vi "SubPanel_DataCollection_Rev11_v14.vi"(0 "DCPowerInformationClusterArray_Input":T6(array[cluster]), 1 "VISAPowerInfoInputArray":T5(array[cluster]), 2 "Run Data SubPanel Input":T4, 3 "RF Block Input Array":T1[](array[typedef]), 4 "Oscilloscope Info Array":T3(array[cluster]) {"vertical coupling" items=["AC", "DC", "Ground"]}, 5 "Plot Color Array":u32[](array[colorbox])=[16711686, 65351, 8978420, 14474240, 16139007, 16752640, 8958719, 16758973, 16777215, 46792, 11992992, 12961221, 16763690, 12600063, 16711835, 2953983, 40796, 13111296, 13352613, 9221011, 12964076, 12819897, 65442, 16776704, 14540253, 16740729, 10658047, 10813344, 16753521, 13413843, 8691115, 10339240, 14401205, 16746704, 7467519, 16775978, 13872558, 11387603, 13354405, 10420227, 13107364, 4060, 35208, 11817216, 7566080, 40796, 7539456, 2837073, 6372186, 7499083, 10648702, 16757152], 6 "New Run?":bool, 7 "error in":errorcluster) -> (20 "DCPowerInformationClusterArray_Output":T6(array[cluster]), 21 "VISAPowerInfoInputOutput":T5(array[cluster]), 22 "Run Data SubPanel Output":T4, 23 "RF Subpanel Output":T1[](array[typedef]), 24 "Oscilloscope Info Array Output":T3(array[cluster]) {"vertical coupling" items=["AC", "DC", "Ground"]}, 25 "Reinitialize?":bool, 26 "Data Was Collected?":bool, 27 "error out":errorcluster)   [LabVIEW 2019]
uses:
  Controls/DataBlockControl.ctl
  Controls/QueueDataControl_V3.ctl
  <vilib>/Utility/file.llb/Write Delimited Spreadsheet (string).vi
  Controls/RFBlockControl.ctl
  <instrlib>/niScope/Controls/niScope vertical coupling.ctl
panel:
  in  "Total Current Y Min":dbl
  in  "Total Current Y Max":dbl
  in  "Total Voltage Y Min":dbl
  in  "Total Voltage Y Max":dbl
  in  "Total Measurement Range Update":bool
  in  "Live Measurement Range Update":bool
  in  "Live Current Y Min":dbl
  in  "Live Current Y Max":dbl
  in  "Live Voltage Y Min":dbl
  in  "Live Voltage Y Max":dbl
  out "Current Measurements Live":cluster{dbl[], dbl[]}[](graph)
  out "Voltage Measurements Live":cluster{dbl[], dbl[]}[](graph)
  out "RFSourceInfoArray":string[][](array[string])
  out "OscilloscopeInfoArray":string[][](array[string])
  out "Voltage Waveform Array":waveform(dbl)[](graph)
  out "Current Waveform Array":waveform(dbl)[](graph)
  out "DCPowerInfoArray":string[][](array[string])
  out "Current Measurements Total":cluster{dbl[], dbl[]}[](graph)
  out "Voltage Measurements Total":cluster{dbl[], dbl[]}[](graph)
  out "Exiting":bool
  out "Full Run Information":string
  out "Ready For Next Run?":bool
  in  "Next Run":bool
  out "Recording Data":bool
  in  "Record Data Toggle":bool
  out "error of collection":errorcluster
  in  "force exit SubVI":bool
  out "RF Block Parameters Output":T1
  # "Background information (Important)\nThere are three sets of voltage/current graphs\n\nOne is live always and just shows what all the channels look like _______ Waveform Array\n\nOne is live when measuring and shows some duration of the recording _______ Measurements Live\n\nOne shows the entire duration of the run, but it will take a few seconds to compile, just be patient it will populate\n\n\nInstructions (More Important)"
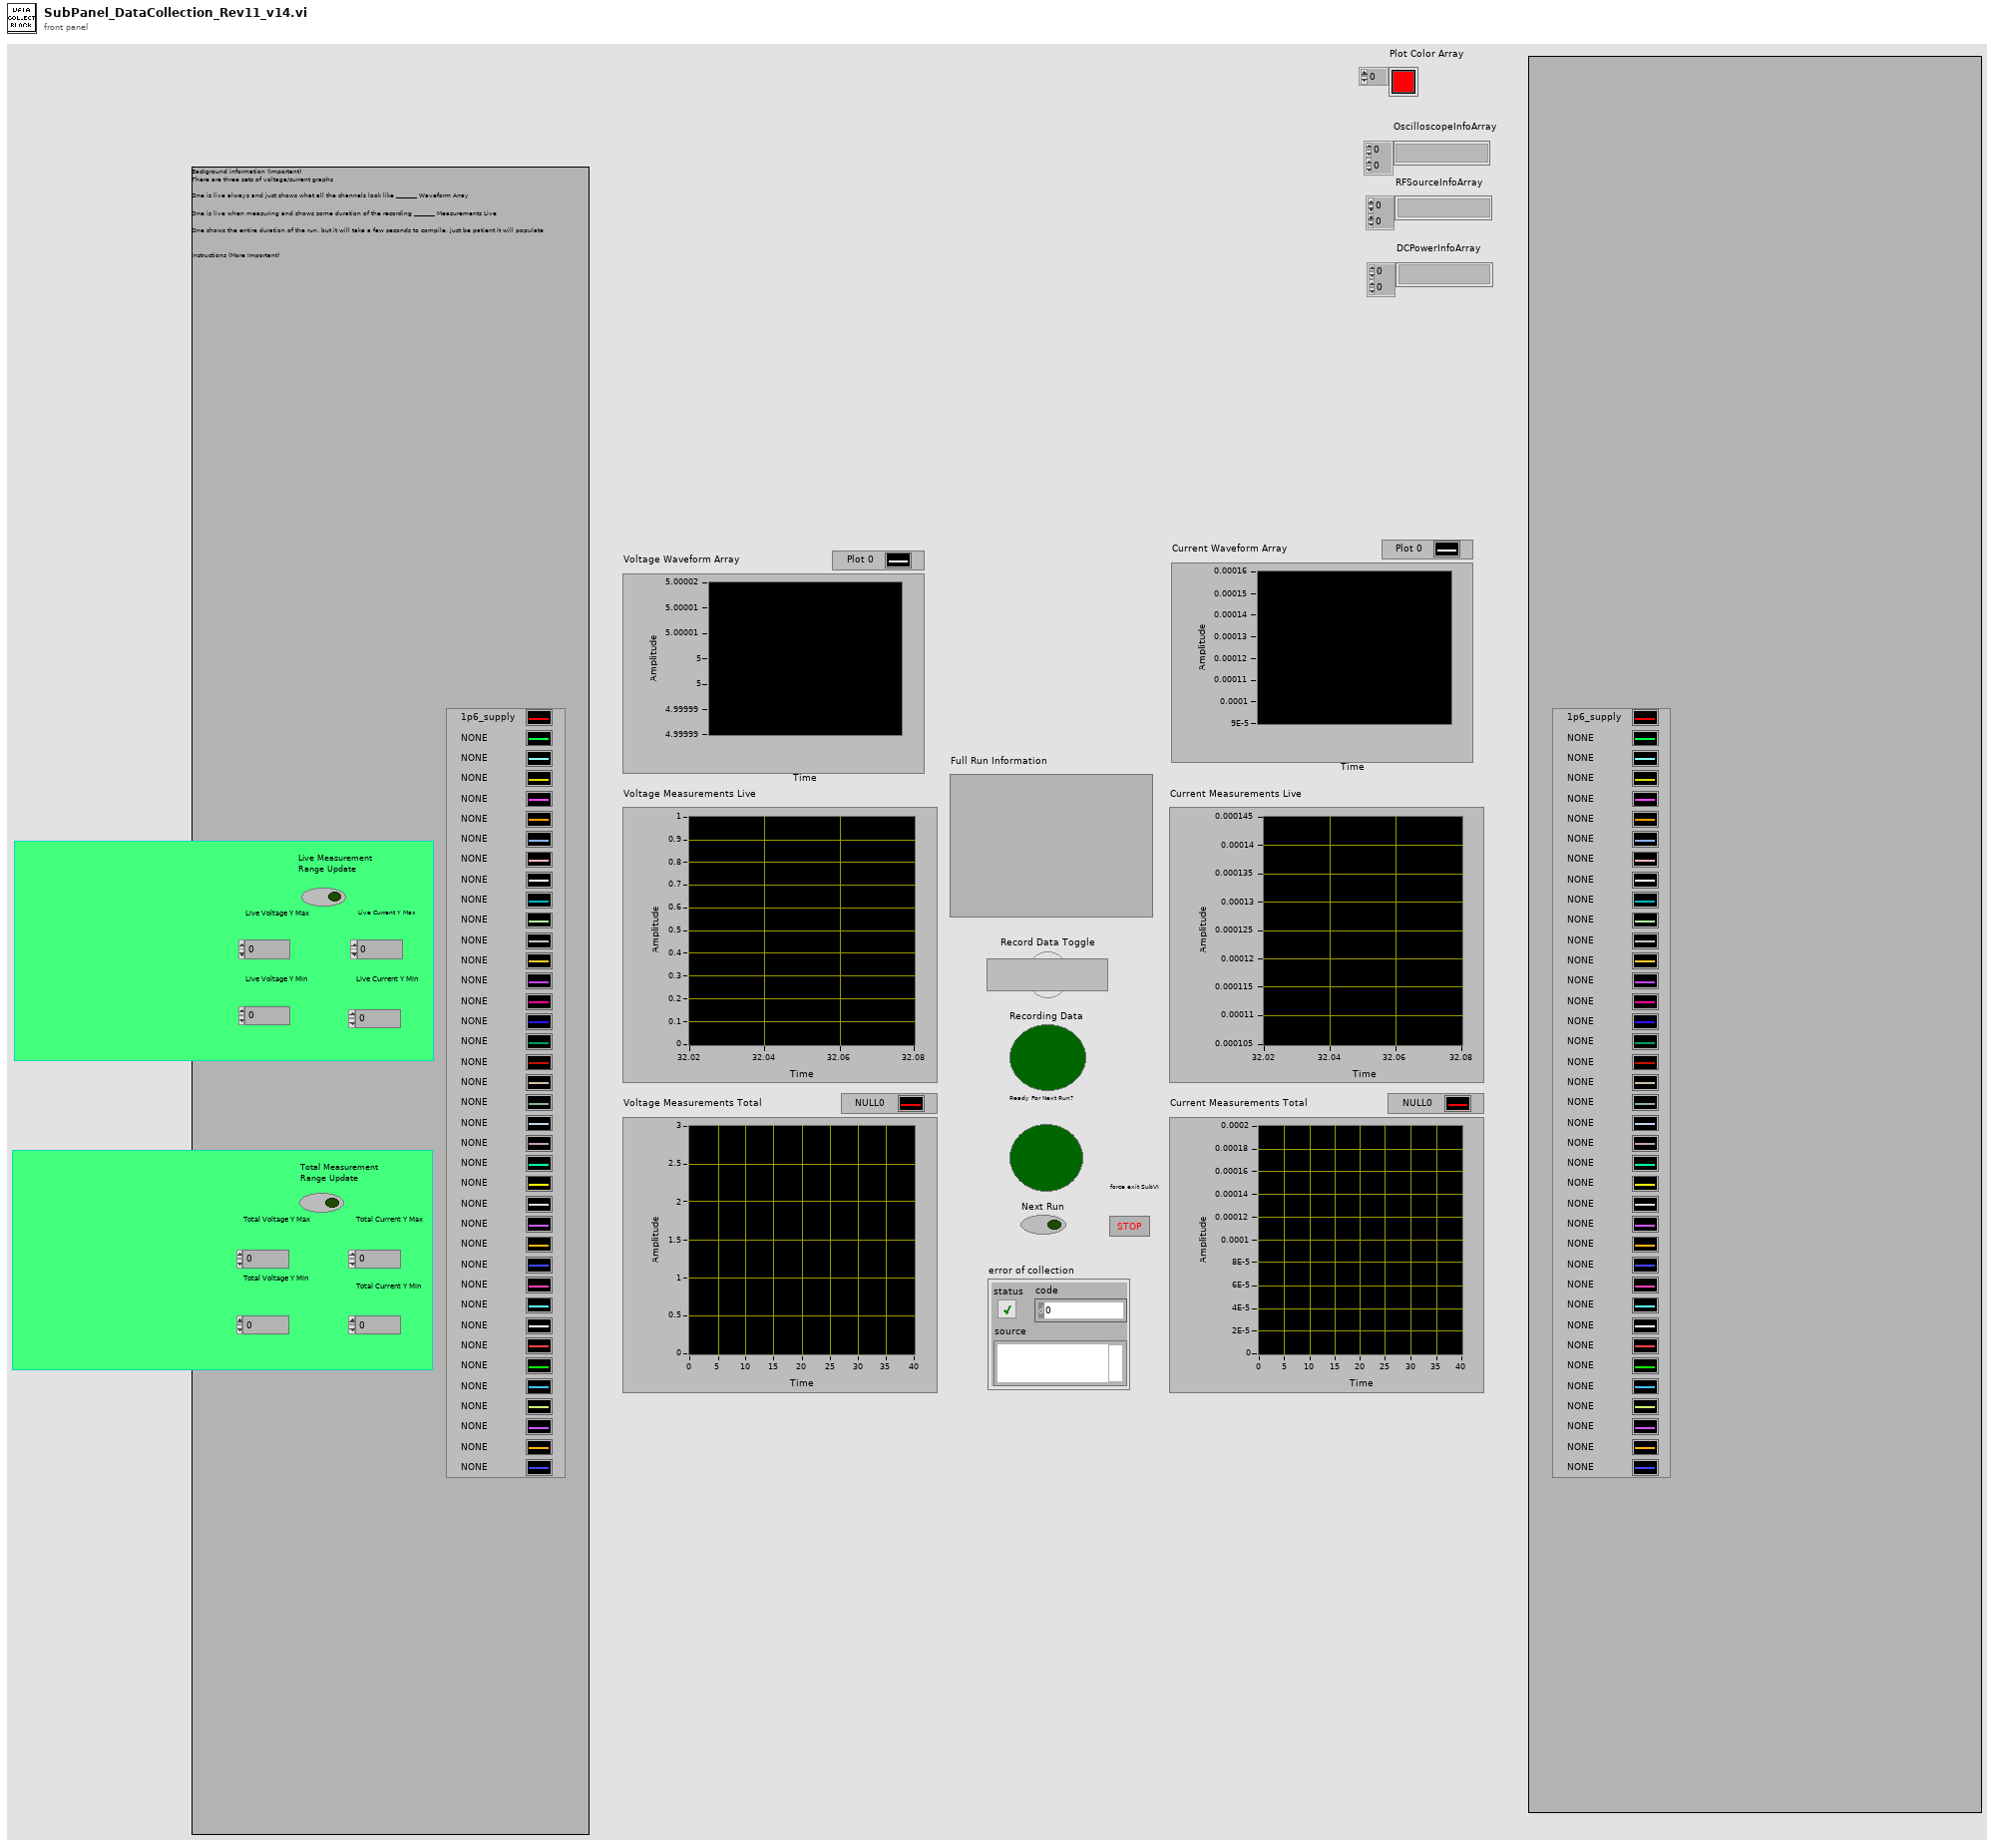
[diagram p1: front panel]
types:
  T1 = typedef "RFBlockControl.ctl" = cluster{"VISA resource name":refnum<visa-resource-name>, "RF Power State In":bool, "Frequency (GHz) Output":dbl, "Power (dBm) Output":dbl, "Instrument Name":string}
  T2 = typedef "niScope vertical coupling.ctl" = i32
  T3 = cluster{"instrument handle out":refnum<k15>, "channel numbers array":string[], "channel names array":string[], "vertical range":dbl, "vertical coupling":T2, "Channel 0 50 ohms?":bool, "50 ohm vertical range (V)":dbl, "min record length":i32, "Actual Sample Rate":dbl}[]
  T4 = typedef "DataBlockControl.ctl" = cluster{"Run Folder Parent Directory":path, "DUT":string, "Ion (ex Kr)":string, "Board Number":string, "Effective LET":string, "Test Type":enum16{"Single Event Latchup", "Single Event Transient", "Single Event Upset"}}
  T5 = cluster{"VISA resource name":refnum<visa-resource-name>, "String List":string, string[], "Input Array (Voltage,Current_Limit)":dbl[], "Input Array (Voltage,Current_Limit)":dbl[], "Channel Names":string[], "read buffer":string}[]
  T6 = cluster{"instrument handle out":refnum<k15>, string, string[], dbl[], string[], "Current Limit Output Array":dbl[], dbl[]}[]
  T7 = typedef "QueueDataControl_V3.ctl" = cluster{"Array of fetched data":dbl[][][], "Channel Names Array":string[], "Voltage Waveform Array":waveform(dbl)[], "Current Waveform Array":waveform(dbl)[], "Resetting Time":timestamp}
  T8 = cluster{"IVI Refnum out":refnum<k15>, string, "voltage level channel 23":dbl, "Channel Name 23":string, "Current Limit":dbl, "Measure Record dt":dbl, string}[]
  T9 = cluster{"created path":path, "DCPowerInformation_byChannel":cluster{"IVI Refnum out":refnum<k15>, string, "voltage level channel 23":dbl, "Channel Name 23":string, "Current Limit":dbl, "Measure Record dt":dbl, string}[], string[]}
  T10 = cluster{"Array of fetched data":dbl[][], string, i32[]}
  T11 = enum16{"open", "replace", "create", "open or create", "replace or create", "replace or create with confirmation"}
  T12 = enum16{"Single Event Latchup", "Single Event Transient", "Single Event Upset"}
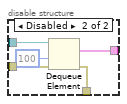
[diagram p5: hidden frame]
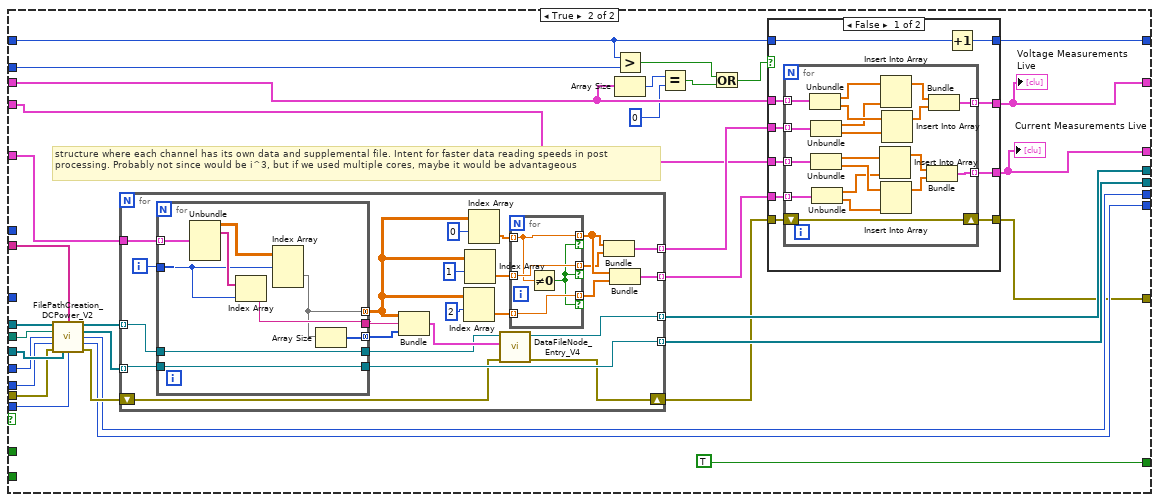
[diagram p7: hidden frame]
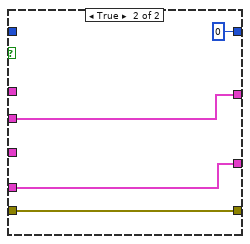
[diagram p8: hidden frame]
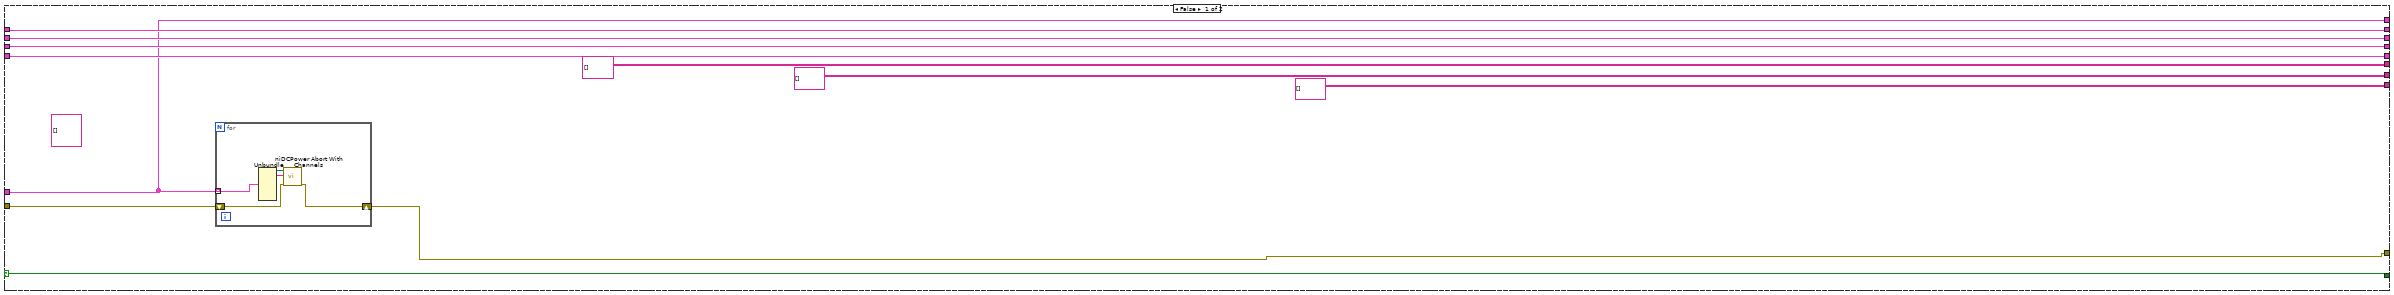
[diagram p9: hidden frame]
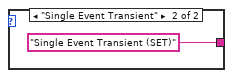
[diagram p10: hidden frame]
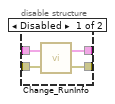
[diagram p14: hidden frame]
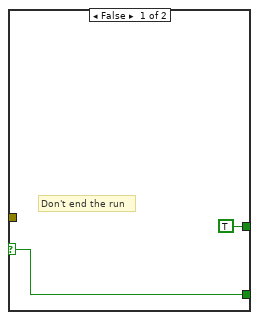
[diagram p17: hidden frame]
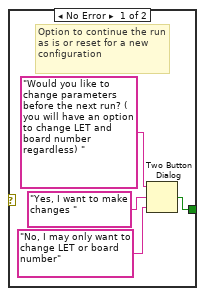
[diagram p18: hidden frame]
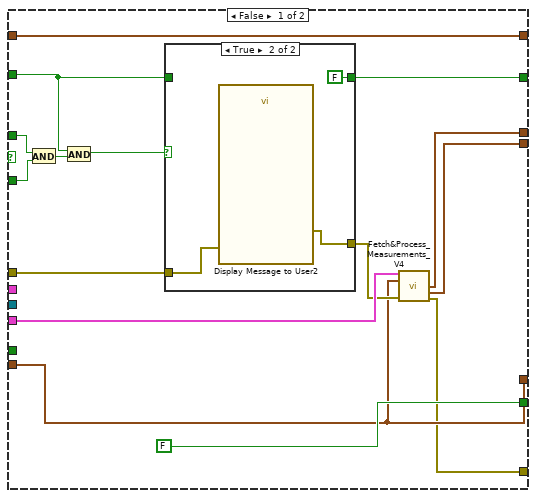
[diagram p20: hidden frame]
diagram:
  w15 = cluster{dbl[], dbl[]}[] [] ("array")
  (unwired) string[] ["Instrument Name", "Channel Name", "Instrument Channel Number", "Voltage (V)", "Current Limit (A)", "Measure Record delta Time (s)"] ("new element/subarray")
  w50 = T7 {"Array of fetched data"=[], "Channel Names Array"=[], "Voltage Waveform Array"=[], "Current Waveform Array"=[], "Resetting Time"=timestamp(0 s since 1904-01-01)} ("DCPower Queue Data Double Array Format")
  (unwired) T7 {"Array of fetched data"=[], "Channel Names Array"=[], "Voltage Waveform Array"=[], "Current Waveform Array"=[], "Resetting Time"=timestamp(0 s since 1904-01-01)} ("DCPower Double Array Queue")
  (unwired) 10000 ("binary file indexor in")
  (unwired) T4 {"Run Folder Parent Directory"=path "", "DUT"="", "Ion (ex Kr)"="", "Board Number"="", "Effective LET"="", "Test Type"=enum."Single Event Latchup"} ("Run Data Configuration")
  # "Need to make a function that will decrease the amount of loops if there are more channels active. Just exponential decay or a X/Y function but need some kind of offset which will probably be experimentally determined"
  # "Initiating the queue"
  # "echoing run information"
  # "Checking if this is a new run. If it is, a new folder is created along with references to a datafile node. If it is not new (i.e. you didn't start recording data because you needed to make a last minute change and pressed forced exit subvi), the previous folder that is theoretically empty (or just has the .txt files is used"
  # "If yes, you go into this subVI"
  # "This is the message at the beginning confirming if you want to make small changes to the program (i.e. LET)"
  # "Parameters from the configuration stage of this program"
  # "Reset the graph that is saving every 10 seconds of data. Every reset the low bound of the ten seconds is"
  # "Need to change to reflect number of channels that are being recorded. Collect this from a parameters file eventually that will be created"
  # "Indicator if the system is ready for another run. Also indicates if data was actually collected"
  # "Resets the system to start recording"
  # "A flag to ensure the warning message shows only once and doesn't lock the system"
  # "Initiating all of the DC Power instruments (doing this here so because we force abort channels in the DCPower setup because buffer overflow issues. Iterating over the instrument array and the active channel list"
  n1 = flat-sequence {
    tunnel: [w90] -> w66
    tunnel: "error in" -> [w80]
    tunnel: [w94] -> w71
    tunnel: "Run Data SubPanel Input" -> [w82]
    frame #0 {
      n2 = disable-structure shown="Enabled" {
        disable-tunnel: w80 -> [w97 w108]
        disable-tunnel: [w106 w108] -> w79
        frame Enabled {
          n3 = property on="Voltage Measurements Live" class="XYGraph (strict)"(error in=w97, "BG Color"=u32 0 ("Plot.Plot Color"), "Plot.Plot Interpolation"=u8 2) -> (error out=w96:errorcluster)  [unwired: 1 in, 1 out]
          n4 = property on="Current Measurements Live" class="XYGraph (strict)"(error in=w96, "BG Color"=u32 0 ("Plot.Plot Color"), "Plot.Plot Interpolation"=u8 2) -> (error out=w95:errorcluster)  [unwired: 1 in, 1 out]
          n5 = property on="Voltage Measurements Total" class="XYGraph (strict)"(error in=w95, "BG Color"=u32 0 ("Plot.Plot Color"), "Plot.Plot Interpolation"=u8 2) -> (error out=w107:errorcluster)  [unwired: 1 in, 1 out]
          n6 = property on="Current Measurements Total" class="XYGraph (strict)"(error in=w107, "BG Color"=u32 0 ("Plot.Plot Color"), "Plot.Plot Interpolation"=u8 2) -> (error out=w106:errorcluster)  [unwired: 1 in, 1 out]
        }
        frame Disabled {
        }
      }
      n7 = local write "Voltage Measurements Total"(cluster{dbl[], dbl[]}[] [] ("Voltage Measurements")) -> ()
      n8 = local write "Current Measurements Total"(cluster{dbl[], dbl[]}[] [] ("Current Measurements")) -> ()
      n9 = local write "Recording Data"(FALSE ("Recording Data")) -> ()
      n10 = local write "Exiting"(FALSE ("Forced Exit")) -> ()
      n11 = call "Convert_RunInfoCluster_2_RunInfoStringList.vi"("error in"=w79, "Run Number"="", "Run Data SubPanel Input"=w82) -> ("error output"=w83:errorcluster, "Run Data Output"=w84:string)
      n12 = call "Display Message to User"("error in (no error)"=w83, "Enable"=TRUE, "Message"=w84) -> ("error out"=w90:errorcluster)  [unwired: 7 in, 1 out]
      n13 = Two Button Dialog(message="Changing the LET?", 1:"No" ("F button name (\"Cancel\")"), 2:"Yes" ("T button name (\"OK\")")) -> (T button?=w94:bool)
    }
  }
  n14 = call "Convert_InstrumentReferenceArray_2_ChannelReferenceArray.vi"("error in (no error)"=w66, "DCPowerInformationClusterArray_Input"="DCPowerInformationClusterArray_Input") -> ("error out"=w65:errorcluster, "DCPowerInformation_byChannel"=w8:T8)
  n15 = case shown="True" w71 {
    tunnel: "Run Data SubPanel Input" -> [w110 w114]
    tunnel: [w110 w113] -> w24
    tunnel: [w109 w112] -> w67
    tunnel: w65 -> [w109 w111]
    frame False {
    }
    frame True {
      n16 = disable-structure shown="Enabled" {
        disable-tunnel: w114 -> [w118 w120]
        disable-tunnel: [w117 w119] -> w113
        disable-tunnel: [w116 w122] -> w112
        disable-tunnel: w111 -> [w115 w121]
        frame Disabled {
          n17 = call "Change_RunInfo.vi"("error in (no error)"=w115, "Run Data SubPanel in"=w118) -> ("error out"=w116:errorcluster, "Run Data SubPanel out"=w117:T4)
        }
        frame Enabled {
          n18 = call "Change_RunInfo_V2.vi"("error in (no error)"=w121, "Run Data SubPanel in"=w120) -> ("error out"=w122:errorcluster, "Run Data SubPanel out"=w119:T4)
        }
      }
    }
  }
  n19 = Unbundle(w24) -> ("Run Folder Parent Directory"=w68:path)  [unwired: 5 out]
  n20 = List Folder(path=w68, error in=w67) -> (folder names=w69:string[], error out=w53:errorcluster)  [unwired: 2 in, 2 out]
  n21 = Array Size(array=w69) -> (size(s)=w56:i32)
  n22 = case shown="True" "New Run?" {
    selector: "New Run?" -> [w124 w127]
    tunnel: [w125 w129] -> w57
    tunnel: w56 -> [w125 w128]
    tunnel: [w124 w127] -> w55
    tunnel: [w123 w126] -> w54
    tunnel: w53 -> [w123 w126]
    frame False {
    }
    frame True {
      n23 = Increment(x=w128) -> (x+1=w129:i32)
    }
  }
  n24 = Number To Decimal String(number=w57) -> (decimal integer string=w60:string)  [unwired: 1 in]
  n25 = Concatenate Strings("Run_", w60) -> (w23:string)
  n26 = Array Size(array=w8) -> (size(s)=w52:i32)
  n27 = call "InitialFileFolderCreation_V2.vi"("New Run?"=w55, "error in (no error)"=w54, "Run Number"=w23, "DCPowerArrayClusterSize"=w52, "base path"=w68) -> ("error out"=w22:errorcluster, "SupplementalDataFileReferenceObjectArray"=w63:refnum<file>[], "DataFileReferenceObjectArray"=w64:refnum<file>[], "created path"=w28:path)  [unwired: 3 in]
  n28 = call "Convert_RunInfoCluster_2_RunInfoStringList.vi"("error in"=w22, "Run Number"=w23, "Run Data SubPanel Input"=w24) -> ("error output"=w21:errorcluster, "Run Data Output"=→"Full Run Information":string)
  n29 = for {
    shift-right: [w130] -> w4
    shift-left: w21 -> [w132]
    tunnel: "DCPowerInformationClusterArray_Input" -> [w134] mode=indexing
    n30 = Unbundle(w134) -> ("instrument handle out"=w131:refnum<k15>, w133:string)  [unwired: 5 out]
    n31 = call <instrlib>:"niDCPower Initiate With Channels.vi"("error in (no error)"=w132, "channel name"=w133, "instrument handle"=w131) -> ("error out"=w130:errorcluster)  [unwired: 7 in, 1 out]
  }
  n32 = for {
    shift-right: [w137] -> w6
    shift-left: w4 -> [w139]
    tunnel: "Plot Color Array" -> [_] mode=indexing
    i -> [w135]
    w136 = "NONE" ("Plot.Plot Name")
    n33 = property on="Current Measurements Live" class="XYGraph (strict)"(error in=w139, "Active Plot"=w135, "Plot.Plot Name"=w136) -> (error out=w138:errorcluster)  [unwired: 1 in, 1 out]
    n34 = property on="Voltage Measurements Live" class="XYGraph (strict)"(error in=w138, "Active Plot"=w135, "Plot.Plot Name"=w136) -> (error out=w137:errorcluster)  [unwired: 1 in, 1 out]
  }
  n35 = case shown="Error .." w6 {
    selector: w6 -> [w140 _]
    tunnel: [w140 w141] -> w5
    tunnel: w4 -> [_ w141]
    frame No Error {
    }
    frame Error {
    }
  }
  n36 = for {
    tunnel: w8 -> [w144] mode=indexing
    tunnel: [w147] -> w9 mode=indexing
    shift-right: [w143] -> w11
    shift-left: w5 -> [w146]
    tunnel: "Plot Color Array" -> [w142] mode=indexing
    i -> [w148]
    # "Creating Array of Channel Names"
    n37 = Unbundle(w144) -> ("Channel Name 23"=w147:string)  [unwired: 6 out]
    n38 = property on="Current Measurements Live" class="XYGraph (strict)"(error in=w146, "Active Plot"=w148, "Plot.Plot Name"=w147, "Plot.Plot Color"=w142) -> (error out=w145:errorcluster)  [unwired: 1 in, 1 out]
    n39 = property on="Voltage Measurements Live" class="XYGraph (strict)"(error in=w145, "Active Plot"=w148, "Plot.Plot Name"=w147, "Plot.Plot Color"=w142) -> (error out=w143:errorcluster)  [unwired: 1 in, 1 out]
  }
  n40 = disable-structure shown="Enabled" {
    disable-tunnel: w11 -> [w152 w154]
    disable-tunnel: [w151 w154] -> w10
    disable-tunnel: [w150 _] -> w12
    disable-tunnel: w50 -> [w149 _]
    frame Enabled {
      n41 = Obtain Queue(name (unnamed)="DCPowerQueue", element data type=w149, error in (no error)=w152) -> (queue out=w150:refnum<queue>, error out=w151:errorcluster)  [unwired: 2 in, 1 out]
    }
    frame Disabled {
    }
  }
  n42 = Bundle("created path"=w28, "DCPowerInformation_byChannel"=w8, w9) -> (w42:T9)  [unwired: 1 in]
  n43 = Array Size(array=w9) -> (size(s)=w14:i32)
  n44 = Get Date/Time In Seconds() -> (seconds since 1Jan1904=w26:timestamp)
  n45 = while {
    tunnel: w12 -> [w194]
    shift-right: [w155] -> w47
    shift-left: w10 -> [w193]
    tunnel: w28 -> [w190]
    shift-right: [w183] -> w49
    shift-left: w64 -> [w191]
    shift-right: [w182] -> w48
    shift-left: w63 -> [w189]
    shift-right: [w185] -> _
    shift-left: 0 ("binary file indexor in") -> [w188]
    shift-right: [w184] -> _
    shift-left: 0 ("binary file indexor in") -> [w187]
    tunnel: 1000 ("binary file indexor in") -> [w186]
    tunnel: w9 -> [w192]
    tunnel: w14 -> [w161]
    shift-right: [w171] -> _
    shift-left: FALSE -> [w170]
    shift-right: [w167] -> _
    shift-left: 0 -> [w168]
    shift-right: [w166] -> _
    shift-left: w15 -> [w163]
    shift-right: [w165] -> _
    shift-left: w15 -> [w164]
    tunnel: 251 ("y") -> [w162]
    tunnel: "Plot Color Array" -> [w160]
    stop <- w179 stop-if-true
    # "If recording data is on, there should always be elements in the queue, so I shouldn't have to worry about a state where the \"recording data\" is active but there is no data in the queue, if so, then I'll just have to find an alternative to the OR statement"
    n46 = Get Queue Status(queue=w194, error in (no error)=w193) -> (queue out=w176:refnum<queue>, error out=w177:errorcluster, # elements in queue=w172:i32)  [unwired: 1 in, 5 out]
    n47 = local read "Recording Data"() -> (w169:bool)
    n48 = disable-structure shown="Enabled" {
      disable-tunnel: [w214 w216] -> w178
      disable-tunnel: w177 -> [w213 w218]
      disable-tunnel: w176 -> [w212 w219]
      disable-tunnel: [w211 w215] -> w175
      frame Enabled {
        n49 = Flush Queue(queue=w212, error in (no error)=w213) -> (remaining elements=w211:T7[], error out=w214:errorcluster)  [unwired: 1 out]
      }
      frame Disabled {
        n50 = Dequeue Element(queue=w219, timeout in ms (-1)=100, error in (no error)=w218) -> (element=w215:T7, error out=w216:errorcluster)  [unwired: 2 out]
      }
    }
    n51 = Not Equal To 0?(x=w172) -> (x != 0?=w174:bool)
    n52 = And(x=w174, y=w169) -> (x .and. y?=w173:bool)
    n53 = case shown="False" w173 {
      tunnel: w175 -> [_ w291]
      tunnel: w178 -> [w229 w285]
      tunnel: w192 -> [w230 w278]
      tunnel: w191 -> [w237 w290]
      tunnel: w190 -> [w231 w289]
      tunnel: w189 -> [w238 w288]
      tunnel: w188 -> [w236 w287]
      tunnel: w187 -> [w235 w277]
      tunnel: w186 -> [_ w276]
      tunnel: [w236 w284] -> w185
      tunnel: [w235 w283] -> w184
      tunnel: [w237 w280] -> w183
      tunnel: [w238 w279] -> w182
      tunnel: [w228 w270] -> w159
      tunnel: [w227 TRUE] -> w171
      tunnel: w170 -> [w226 _]
      tunnel: w169 -> [w234 _]
      tunnel: w168 -> [w225 w268]
      tunnel: [w224 w267] -> w167
      tunnel: [w223 w274] -> w166
      tunnel: [w222 w271] -> w165
      tunnel: w164 -> [w222 w266]
      tunnel: w163 -> [w223 w265]
      tunnel: w162 -> [_ w259]
      tunnel: w161 -> [w221 _]
      tunnel: w160 -> [w220 _]
      frame False {
        n54 = Not(x=w234) -> (.not. x?=w233:bool)
        n55 = And(x=w233, y=w226) -> (x .and. y?=w232:bool)
        n56 = case shown="True" w232 {
          tunnel: w231 -> [_ w253]
          tunnel: w230 -> [_ w252]
          tunnel: w229 -> [w241 w245]
          tunnel: [w241 w250] -> w228
          tunnel: [w240 FALSE] -> w227
          tunnel: w226 -> [w240 _]
          tunnel: w225 -> [w239 _]
          tunnel: [w239 0] -> w224
          tunnel: w221 -> [_ w243]
          tunnel: w220 -> [_ w242]
          frame False {
          }
          frame True {
            n57 = for {
              N: w243 -> [_]
              shift-right: [w256] -> w244
              shift-left: w245 -> [w257]
              tunnel: w242 -> [w254] mode=indexing
              i -> [w255]
              n58 = property on="Current Measurements Total" class="XYGraph (strict)"(error in=w257, "Active Plot"=w255, "Plot.Plot Color"=w254) -> (error out=w258:errorcluster)  [unwired: 1 in, 1 out]
              n59 = property on="Voltage Measurements Total" class="XYGraph (strict)"(error in=w258, "Active Plot"=w255, "Plot.Plot Color"=w254) -> (error out=w256:errorcluster)  [unwired: 1 in, 1 out]
            }
            n60 = call "ReadDataFile_V1.vi"("error in (no error)"=w244, "Create CSV files?"=FALSE, "Channel Names Array"=w252, "DataFolder Path"=w253) -> ("error out"=w250:errorcluster, "Current Measurements"=→"Current Measurements Total":cluster{dbl[], dbl[]}[], "Voltage Measurements"=→"Voltage Measurements Total":cluster{dbl[], dbl[]}[])  [unwired: 5 in]
          }
        }
      }
      frame True {
        # "structure where each channel has its own data and supplemental file. Intent for faster data reading speeds in post processing. Probably not since would be i^3, but if we used multiple cores, maybe it would be advantageous"
        n61 = call "FilePathCreation_DCPower_V2.vi"("binary file input reference array 1"=w290, "Channel Name Input array"=w278, "data output directory folder"=w289, "binary file indexor in"=w287, "Reset counter in"=w277, "error in (no error)"=w285, "binary file input reference array 2"=w288, "reset threshold"=w276) -> ("binary file output reference array"=w282:refnum<file>[], "binary file output reference array 2"=w281:refnum<file>[], "binary file indexor out"=w284:i32, "reset counter out"=w283:i32, "error out"=w286:errorcluster)  [unwired: 3 in]
        n62 = for {
          shift-right: [w338] -> w269
          shift-left: w286 -> [w339]
          tunnel: w291 -> [w348]
          tunnel: w281 -> [w345] mode=indexing
          tunnel: w282 -> [w344] mode=indexing
          tunnel: [w343] -> w279 mode=indexing
          tunnel: [w337] -> w280 mode=indexing
          tunnel: [w326] -> w273 mode=indexing
          tunnel: [w325] -> w272 mode=indexing
          i -> [w342]
          n63 = for {
            tunnel: w348 -> [w361] mode=indexing
            tunnel: w342 -> [w358]
            tunnel: [w353] -> w333 mode=concatenating
            tunnel: [w357] -> w347
            tunnel: w345 -> [w356]
            tunnel: w344 -> [w354]
            tunnel: [w354] -> w340
            tunnel: [w356] -> w343
            tunnel: [w355] -> w346 mode=concatenating
            n64 = Unbundle(w361) -> ("Array of fetched data"=w360:dbl[][][], "Channel Names Array"=w359:string[])  [unwired: 3 out]
            n65 = Index Array(array=w359, index=w358) -> (element=w357:string)
            n66 = Index Array(array=w360, index (dim 0)=w358) -> (element=w353:dbl[][])  [unwired: 2 in]
            n67 = Array Size(array=w353) -> (size(s)=w355:i32[])
          }
          n68 = Bundle("Array of fetched data"=w333, w347, w346) -> (w341:T10)  [unwired: 1 in]
          n69 = Index Array(array=w333, index (row)=2) -> (element=w330:dbl[])  [unwired: 1 in]
          n70 = Index Array(array=w333, index (row)=1) -> (element=w331:dbl[])  [unwired: 1 in]
          n71 = Index Array(array=w333, index (row)=0) -> (element=w332:dbl[])  [unwired: 1 in]
          n72 = call "DataFileNode_Entry_V4.vi"("error in (no error)"=w339, "Queued Elements"=w341, "Byte Stream File in"=w340) -> ("error out"=w338:errorcluster, "Byte Stream File out"=w337:refnum<file>)  [unwired: 7 in]
          n73 = for {
            tunnel: [w350] -> w329 mode=indexing if=w349
            tunnel: w332 -> [w350] mode=indexing
            tunnel: [w352] -> w327 mode=indexing if=w349
            tunnel: w331 -> [w352] mode=indexing
            tunnel: [w351] -> w328 mode=indexing if=w349
            tunnel: w330 -> [w351] mode=indexing
            n74 = Not Equal To 0?(x=w350) -> (x != 0?=w349:bool)
          }
          n75 = Bundle(w329, w327) -> (w326:cluster{dbl[], dbl[]})  [unwired: 1 in]
          n76 = Bundle(w329, w328) -> (w325:cluster{dbl[], dbl[]})  [unwired: 1 in]
        }
        n77 = Greater?(x=w268, y=w259) -> (0:w261:bool)
        n78 = Array Size(array=w265) -> (size(s)=w264:i32)
        n79 = Equal?(x=w264, y=0) -> (x = y?=w262:bool)
        n80 = Or(x=w261, y=w262) -> (x .or. y?=w260:bool)
        n81 = case shown="False" w260 {
          tunnel: [w297 w321] -> w274
          tunnel: w265 -> [w301 _]
          tunnel: w273 -> [w300 w321]
          tunnel: w266 -> [w299 _]
          tunnel: w272 -> [w298 w322]
          tunnel: [w296 w322] -> w271
          tunnel: [w295 w324] -> w270
          tunnel: w269 -> [w294 w324]
          tunnel: w268 -> [w293 _]
          tunnel: [w292 0] -> w267
          frame False {
            n82 = for {
              tunnel: w301 -> [w320] mode=indexing
              tunnel: w300 -> [w317] mode=indexing
              tunnel: w299 -> [w314] mode=indexing
              tunnel: w298 -> [w313] mode=indexing
              tunnel: [w304] -> w297 mode=indexing
              tunnel: [w303] -> w296 mode=indexing
              shift-right: [w302] -> w295
              shift-left: w294 -> [w302]
              n83 = Unbundle(w320) -> (w319:dbl[], w318:dbl[])
              n84 = Unbundle(w317) -> (w316:dbl[], w315:dbl[])
              n85 = Unbundle(w314) -> (w312:dbl[], w311:dbl[])
              n86 = Unbundle(w313) -> (w310:dbl[], w309:dbl[])
              n87 = Insert Into Array(array=w312, new element=w310) -> (w307:dbl[])  [unwired: 1 in]
              n88 = Insert Into Array(array=w319, new element=w316) -> (w305:dbl[])  [unwired: 1 in]
              n89 = Insert Into Array(array=w311, new element=w309) -> (w308:dbl[])  [unwired: 1 in]
              n90 = Insert Into Array(array=w318, new element=w315) -> (w306:dbl[])  [unwired: 1 in]
              n91 = Bundle(w307, w308) -> (w303:cluster{dbl[], dbl[]})  [unwired: 1 in]
              n92 = Bundle(w305, w306) -> (w304:cluster{dbl[], dbl[]})  [unwired: 1 in]
            }
            n93 = Increment(x=w293) -> (x+1=w292:i32)
          }
          frame True {
          }
        }
        "Voltage Measurements Live" <- w274
        "Current Measurements Live" <- w271
      }
    }
    n94 = local read "Exiting"() -> (w181:bool)
    n95 = Equal To 0?(x=w172) -> (x = 0?=w180:bool)
    n96 = case shown="True" "Live Measurement Range Update" {
      tunnel: w159 -> [w203 w210]
      tunnel: [w203 w208] -> w156
      frame False {
      }
      frame True {
        n97 = property on="Voltage Measurements Live" class="XYGraph (strict)"(error in=w210, "YScale.Maximum"="Live Voltage Y Max", "YScale.Minimum"="Live Voltage Y Min") -> (error out=w209:errorcluster)  [unwired: 1 in, 1 out]
        n98 = property on="Current Measurements Live" class="XYGraph (strict)"(error in=w209, "YScale.Maximum"="Live Current Y Max", "YScale.Minimum"="Live Current Y Min") -> (error out=w208:errorcluster)  [unwired: 1 in, 1 out]
      }
    }
    n99 = And(x=w180, y=w181) -> (x .and. y?=w179:bool)
    n100 = case shown="True" "Total Measurement Range Update" {
      tunnel: w156 -> [w195 w202]
      tunnel: [w195 w200] -> w155
      frame False {
      }
      frame True {
        n101 = property on="Voltage Measurements Total" class="XYGraph (strict)"(error in=w202, "YScale.Maximum"="Total Voltage Y Max", "YScale.Minimum"="Total Voltage Y Min") -> (error out=w201:errorcluster)  [unwired: 1 in, 1 out]
        n102 = property on="Current Measurements Total" class="XYGraph (strict)"(error in=w201, "YScale.Maximum"="Total Current Y Max", "YScale.Minimum"="Total Current Y Min") -> (error out=w200:errorcluster)  [unwired: 1 in, 1 out]
      }
    }
  }
  n103 = while {
    shift-right: [w392] -> w32
    shift-left: "DCPowerInformationClusterArray_Input" -> [w392]
    shift-right: [w396] -> w34
    shift-left: "VISAPowerInfoInputArray" -> [w396]
    shift-right: [w395] -> w36
    shift-left: w24 -> [w395]
    shift-right: [w394] -> w38
    shift-left: "RF Block Input Array" -> [w394]
    shift-right: [w393] -> w40
    shift-left: "Oscilloscope Info Array" -> [w393]
    shift-right: [w362] -> w51
    shift-left: w10 -> [w390]
    tunnel: w8 -> [w391]
    shift-right: [w389] -> _
    shift-left: FALSE -> [w386]
    tunnel: w12 -> [w388]
    shift-right: [w372] -> _
    shift-left: FALSE -> [w377]
    tunnel: [w381] -> w75
    shift-right: [w375] -> _
    shift-left: TRUE ("x .and. y?") -> [w376]
    shift-right: [w373] -> _
    shift-left: w26 -> [w374]
    tunnel: [w372] -> w31
    tunnel: w50 -> [w370]
    shift-right: [w367] -> w1
    shift-left: timestamp(0 s since 1904-01-01) ("seconds since 1Jan1904") -> [w366]
    stop <- w371 stop-if-true
    # "If I am going to reset the entire configuration or if we are going up in LET only. True, reset the system. False, don't reset the system"
    n104 = Not(x=w377) -> (.not. x?=w379:bool)
    n105 = And(x="Record Data Toggle", y=w379) -> (x .and. y?=w380:bool)
    "Recording Data" <- w380
    n106 = case shown="True" w380 {
      tunnel: w391 -> [w425 w440]
      tunnel: w390 -> [w423 w447]
      tunnel: [w413 w435] -> w369
      tunnel: [w414 w434] -> w368
      tunnel: w386 -> [_ w445]
      tunnel: [FALSE w446] -> w389
      tunnel: w388 -> [_ w444]
      tunnel: [w412 w443] -> w384
      tunnel: "Record Data Toggle" -> [w420 _]
      tunnel: w377 -> [w421 _]
      tunnel: w376 -> [w416 _]
      tunnel: [w417 TRUE] -> w375
      tunnel: w374 -> [w415 w448]
      tunnel: [w415 w438] -> w373
      tunnel: w370 -> [_ w442]
      tunnel: [w411 w432] -> w367
      tunnel: w366 -> [w411 w431]
      frame False {
        n107 = And(x=w420, y=w421) -> (x .and. y?=w419:bool)
        n108 = And(x=w416, y=w419) -> (x .and. y?=w418:bool)
        n109 = case shown="True" w418 {
          tunnel: [w427 w429] -> w422
          tunnel: w423 -> [w427 w430]
          tunnel: [w426 FALSE] -> w417
          tunnel: w416 -> [w426 _]
          frame False {
          }
          frame True {
            n110 = call "Display Message to User2"("error in (no error)"=w430) -> ("error out"=w429:errorcluster)  [unwired: 9 in, 1 out]
          }
        }
        n111 = call "Fetch&Process_Measurements_V4.vi"("DCPowerInformation_byChannel"=w425, "Initial Time"=w415, "error in (no error)"=w422) -> ("Current Waveform Array"=w413:waveform(dbl)[], "Voltage Waveform Array"=w414:waveform(dbl)[], "error out"=w412:errorcluster)  [unwired: 6 in, 4 out]
      }
      frame True {
        n112 = case shown="True" w445 {
          tunnel: [w450 w456] -> w438
          tunnel: w448 -> [_ w456]
          tunnel: w447 -> [w451 w455]
          tunnel: [w451 w455] -> w439
          tunnel: [TRUE w454] -> w446
          tunnel: w445 -> [_ w454]
          tunnel: [w450 w453] -> w432
          tunnel: w431 -> [_ w453]
          frame False {
            n113 = Get Date/Time In Seconds() -> (seconds since 1Jan1904=w450:timestamp)
          }
          frame True {
          }
        }
        n114 = call "Fetch&Process_Measurements_V4.vi"("DCPowerInformation_byChannel"=w440, "Initial Time"=w438, "error in (no error)"=w439) -> ("Data As dbl Array"=w437:dbl[][][], "Channel Number Array"=w436:string[], "Current Waveform Array"=w435:waveform(dbl)[], "Voltage Waveform Array"=w434:waveform(dbl)[], "error out"=w433:errorcluster)  [unwired: 6 in, 2 out]
        n115 = Bundle(cluster=w442, "Array of fetched data"=w437, "Channel Names Array"=w436) -> (w441:T7)  [unwired: 3 in]
        n116 = Enqueue Element(queue=w444, element=w441, error in (no error)=w433) -> (error out=w443:errorcluster)  [unwired: 1 in, 2 out]
      }
    }
    "Current Waveform Array" <- w369
    "Voltage Waveform Array" <- w368
    n117 = Not(x=w380) -> (.not. x?=w387:bool)
    n118 = And(x=w387, y=w386) -> (x .and. y?=w385:bool)
    n119 = case shown="True" w385 {
      tunnel: w384 -> [w407 w409]
      tunnel: [w408 TRUE] -> w372
      tunnel: w377 -> [w408 _]
      tunnel: [w407 w409] -> w362
      frame False {
      }
      frame True {
      }
    }
    "error of collection" <- w362
    "Ready For Next Run?" <- w372
    n120 = And(x="Next Run", y=w372) -> (x .and. y?=w383:bool)
    n121 = Or(x="force exit SubVI", y=w383) -> (x .or. y?=w364:bool)
    n122 = Or(x=w362, y=w364) -> (x .or. y?=w363:bool)
    n123 = case shown="True" w363 {
      selector: w363 -> [w398 _]
      tunnel: w362 -> [_ w401]
      tunnel: [w398 TRUE] -> w371
      tunnel: [TRUE ("T button?") w399] -> w381
      frame False {
        # "Don't end the run"
      }
      frame True {
        n124 = case shown="Error .." w401 {
          tunnel: [w402 TRUE] -> w399
          frame No Error {
            # "Option to continue the run as is or reset for a new configuration"
            n125 = Two Button Dialog(message="Would you like to change parameters before the next run? ( you will have an option to change LET and board number regardless) ", 1:"No, I may only want to change LET or board number" ("F button name (\"Cancel\")"), 2:"Yes, I want to make changes " ("T button name (\"OK\")")) -> (T button?=w402:bool)
          }
          frame Error {
            # "End the run immediately. There is an error or an immediate issue with the VI"
          }
        }
      }
    }
    "Exiting" <- w371
  }
  "Reinitialize?" <- w75
  n126 = for {
    tunnel: w49 -> [w461] mode=indexing
    tunnel: w48 -> [w459] mode=indexing
    shift-right: [w457] -> w46
    shift-left: w47 -> [w460]
    n127 = Close File(refnum=w461, error in=w460) -> (error out=w458:errorcluster)  [unwired: 1 out]
    n128 = Close File(refnum=w459, error in=w458) -> (error out=w457:errorcluster)  [unwired: 1 out]
  }
  n129 = Merge Errors(w51, w46) -> (w43:errorcluster)
  n130 = Unbundle(w42) -> ("created path"=w3:path)  [unwired: 2 out]
  n131 = case shown="True" w31 {
    selector: w31 -> [w468 w608]
    tunnel: w43 -> [w463 w614]
    tunnel: [w472 w546] -> w41
    tunnel: w40 -> [w472 w613]
    tunnel: [w471 w548] -> w39
    tunnel: w38 -> [w471 w612]
    tunnel: [w470 w534] -> w37
    tunnel: w36 -> [w470 w611]
    tunnel: [w469 w551] -> w35
    tunnel: w34 -> [w469 w610]
    tunnel: [w464 w553] -> w33
    tunnel: w32 -> [w464 w609]
    tunnel: [w468 w608] -> w30
    tunnel: [string[][] [] ("DCPowerInfoArray") w544] -> w29
    tunnel: w3 -> [_ w479]
    tunnel: [string[][] [] ("DCPowerInfoArray") w542] -> w18
    tunnel: [string[][] [] ("DCPowerInfoArray") w536] -> w17
    tunnel: [w462 w481] -> w2
    tunnel: w1 -> [_ w480]
    frame False {
      (unwired) string[][][] []
      n132 = for {
        tunnel: w464 -> [w475] mode=indexing
        shift-right: [w476] -> w462
        shift-left: w463 -> [w477]
        n133 = Unbundle(w475) -> ("instrument handle out"=w474:refnum<k15>, w473:string)  [unwired: 5 out]
        n134 = call <instrlib>:"niDCPower Abort With Channels.vi"("error in (no error)"=w477, "channel name"=w473, "instrument handle"=w474) -> ("error out"=w476:errorcluster)  [unwired: 7 in, 1 out]
      }
    }
    frame True {
      # "This will be indexed eventually"
      n135 = for {
        shift-right: [w707] -> w478
        shift-left: w614 -> [w719]
        tunnel: w609 -> [w710] mode=indexing
        shift-right: [w718] -> w584
        shift-left: w613 -> [w718]
        shift-right: [w717] -> w583
        shift-left: w612 -> [w717]
        shift-right: [w716] -> w582
        shift-left: w611 -> [w716]
        shift-right: [w715] -> w581
        shift-left: w610 -> [w715]
        shift-right: [w714] -> w580
        shift-left: w609 -> [w714]
        shift-right: [w712] -> w585
        shift-left: string[][] [] ("DCPowerInfoArray") -> [w713]
        # "This puts all the instruments together in one output"
        n136 = Unbundle(w710) -> ("instrument handle out"=w721:refnum<k15>, w720:string)  [unwired: 5 out]
        n137 = call <instrlib>:"niDCPower Abort With Channels.vi"("error in (no error)"=w719, "channel name"=w720, "instrument handle"=w721) -> ("error out"=w708:errorcluster)  [unwired: 7 in, 1 out]
        n138 = call "DCPower_ParameterCreation.vi"("error in"=w708, "Precision"="8", "DCPowerInformationByInstrument"=w710) -> ("error out"=w707:errorcluster, "DCPowerInfoArray"=w706:string[][])
        n139 = Insert Into Array(array=w713, index (col)=0 ("disabled index (col)"), new element=w706) -> (w712:string[][])  [unwired: 1 in]
      }
      n140 = Concatenate Strings("Channel Name " ("string")) -> (w597:string)
      n141 = Concatenate Strings("Voltage (V) " ("string")) -> (w599:string)
      n142 = Concatenate Strings("Measure Record delta Time (s) " ("string")) -> (w601:string)
      n143 = Concatenate Strings("Instrument Name " ("string")) -> (w596:string)
      n144 = Concatenate Strings("Instrument Channel Number " ("string")) -> (w598:string)
      n145 = Concatenate Strings("Current Limit (A) " ("string")) -> (w600:string)
      n146 = Build Array(w596, w597, w598, w599, w600, w601) -> (w589:string[])
      n147 = Build Path(base path=w479, name or relative path="DCPOW_Params.csv") -> (appended path=w604:path)
      n148 = Insert Into Array(array=w585, index (col)=0 ("disabled index (col)"), new element=w589) -> (w588:string[][])  [unwired: 1 in]
      n149 = call-poly <vilib>:"Write Delimited Spreadsheet.vi"("file path (dialog if empty)"=w604, "format (%s)"="%s" ("format (%.3f)"), "2D data"=w588, "error in (no error)"=w478, "transpose? (no:F)"=TRUE, "delimiter (\\t)"="," ("delimiter (\\t)")) -> ("error out"=w586:errorcluster)  [unwired: 8 in, 1 out]
      n150 = for {
        shift-right: [w700] -> w566
        shift-left: w586 -> [w700]
        shift-right: [w695] -> w554
        shift-left: w580 -> [w695]
        shift-right: [w696] -> w552
        shift-left: w581 -> [w696]
        shift-right: [w697] -> w550
        shift-left: w582 -> [w697]
        shift-right: [w698] -> w549
        shift-left: w583 -> [w698]
        shift-right: [w699] -> w545
        shift-left: w585 -> [w699]
        tunnel: w584 -> [w694] mode=indexing
        tunnel: [w694] -> w547 mode=indexing
        shift-right: [w663] -> w543
        shift-left: string[][] [] ("DCPowerInfoArray") -> [w669]
        n151 = Unbundle(w694) -> ("instrument handle out"=w693:refnum<k15>, "channel numbers array"=w666:string[], "channel names array"=w667:string[], "vertical range"=w688:dbl, "vertical coupling"=w682:T2, "Channel 0 50 ohms?"=w687:bool, "50 ohm vertical range (V)"=w686:dbl, "min record length"=w681:i32, "Actual Sample Rate"=w680:dbl)
        n152 = Array Size(array=w666) -> (size(s)=w689:i32)
        n153 = Initialize Array(w688, w689) -> (w685:dbl[])
        n154 = Decimal String To Number(string="8") -> (number=w664:i32)  [unwired: 2 in, 1 out]
        n155 = case shown="True" w687 {
          tunnel: w686 -> [_ w703]
          tunnel: w685 -> [w701 w705]
          tunnel: [w701 w702] -> w684
          frame False {
          }
          frame True {
            n156 = Replace Array Subset(array=w705, new element=w703, index=0) -> (w702:dbl[])
          }
        }
        n157 = Number To Fractional String(number=w680, precision (6)=w664) -> (F-format string=w674:string)  [unwired: 2 in]
        n158 = Number To Decimal String(number=w681) -> (decimal integer string=w675:string)  [unwired: 1 in]
        n159 = Concatenate Strings(w693) -> (w691:string)
        n160 = Number To Fractional String(number=w684, precision (6)=w664) -> (F-format string=w683:string[])  [unwired: 2 in]
        n161 = Number To Decimal String(number=w682) -> (decimal integer string=w676:string)  [unwired: 1 in]
        n162 = Array Size(array=w666) -> (size(s)=w692:i32)
        n163 = Initialize Array(w691, w692) -> (w690:string[])
        n164 = Array Size(array=w666) -> (size(s)=w679:i32)
        n165 = Array Size(array=w666) -> (size(s)=w677:i32)
        n166 = Array Size(array=w666) -> (size(s)=w678:i32)
        n167 = Initialize Array(w676, w679) -> (w673:string[])
        n168 = Initialize Array(w674, w677) -> (w671:string[])
        n169 = Initialize Array(w675, w678) -> (w672:string[])
        n170 = Build Array(w690, w667, w666, w683, w673, w672, w671) -> (w668:string[][])
        n171 = Insert Into Array(array=w669, index (col)=0 ("disabled index (col)"), new element=w668) -> (w663:string[][])  [unwired: 1 in]
      }
      n172 = Build Array("Instrument Name " ("string"), "Channel Name" ("element"), "Instrument Channel Number" ("element"), "Vertical Range (V)" ("element"), "Vertical Coupling" ("element"), "Min Record Length" ("element"), "Actual Sample Rate" ("element")) -> (w570:string[])
      n173 = Insert Into Array(array=w543, index (col)=0 ("disabled index (col)"), new element=w570) -> (w563:string[][])  [unwired: 1 in]
      n174 = Build Path(base path=w479, name or relative path="Oscilloscope_Params.csv") -> (appended path=w568:path)
      n175 = call-poly <vilib>:"Write Delimited Spreadsheet.vi"("file path (dialog if empty)"=w568, "format (%s)"="%s" ("format (%.3f)"), "2D data"=w563, "error in (no error)"=w566, "transpose? (no:F)"=TRUE, "delimiter (\\t)"="," ("delimiter (\\t)")) -> ("error out"=w561:errorcluster)  [unwired: 8 in, 1 out]
      n176 = for {
        shift-right: [w645] -> w559
        shift-left: string[][] [] ("DCPowerInfoArray") -> [w646]
        tunnel: w549 -> [w661] mode=indexing
        shift-right: [w630] -> w535
        shift-left: w561 -> [w637]
        shift-right: [w638] -> w542
        shift-left: w543 -> [w638]
        shift-right: [w639] -> w544
        shift-left: w545 -> [w639]
        shift-right: [w640] -> w546
        shift-left: w547 -> [w640]
        shift-right: [w641] -> w548
        shift-left: w549 -> [w641]
        shift-right: [w642] -> w534
        shift-left: w550 -> [w642]
        shift-right: [w643] -> w551
        shift-left: w552 -> [w643]
        shift-right: [w644] -> w553
        shift-left: w554 -> [w644]
        n177 = Unbundle(w661) -> ("VISA resource name"=w660:refnum<visa-resource-name>, "Frequency (GHz) Output"=w654:dbl, "Power (dBm) Output"=w651:dbl)  [unwired: 2 out]
        n178 = Decimal String To Number(string="8") -> (number=w649:i32)  [unwired: 2 in, 1 out]
        n179 = VISA Write(VISA resource name=w660, write buffer="*IDN?", error in (no error)=w637) -> (VISA resource name out=w656:refnum<visa-resource-name>, return count=w658:u32, error out=w662:errorcluster)
        n180 = Number To Fractional String(number=w651, precision (6)=w649) -> (F-format string=w652:string)  [unwired: 2 in]
        n181 = Add(x=w658, y=u32 10) -> (x+y=w655:u32)
        n182 = Number To Fractional String(number=w654, precision (6)=w649) -> (F-format string=w653:string)  [unwired: 2 in]
        n183 = VISA Read(VISA resource name=w656, byte count=w655, error in (no error)=w662) -> (read buffer=w636:string, error out=w631:errorcluster)  [unwired: 2 out]
        n184 = Search and Replace String(replace all?=TRUE ("replace all? (F)"), input string=w636, search string=",", replace string="_" ("replace string (\"\")"), error in=w631) -> (result string=w633:string, error out=w630:errorcluster)  [unwired: 3 in, 2 out]
        n185 = Build Array(w633, w653, w652) -> (w648:string[])
        n186 = Insert Into Array(array=w646, index (col)=0 ("index (row)"), new element=w648) -> (w645:string[][])  [unwired: 1 in]
      }
      n187 = Build Array("Instrument Name", "Frequency (GHz)" ("element"), "Power (dBm)" ("element")) -> (w555:string[])
      n188 = Build Path(base path=w479, name or relative path="RFSource_Params.csv") -> (appended path=w540:path)
      n189 = Insert Into Array(array=w559, index (col)=0 ("disabled index (col)"), new element=w555) -> (w536:string[][])  [unwired: 1 in]
      n190 = call-poly <vilib>:"Write Delimited Spreadsheet.vi"("file path (dialog if empty)"=w540, "format (%s)"="%s" ("format (%.3f)"), "2D data"=w536, "error in (no error)"=w535, "transpose? (no:F)"=TRUE, "delimiter (\\t)"="," ("delimiter (\\t)")) -> ("error out"=w515:errorcluster)  [unwired: 8 in, 1 out]
      n191 = Strip Path(path=w479) -> (name=w533:string)  [unwired: 1 out]
      n192 = Unbundle(w534) -> ("DUT"=w532:string, "Ion (ex Kr)"=w531:string, "Board Number"=w530:string, "Effective LET"=w529:string, "Test Type"=w528:T12)  [unwired: 1 out]
      n193 = case shown="\"Single Event Latchup\", Default" w528 {
        tunnel: ["Single Event Latchup (SEL)" "Single Event Transient (SET)"] -> w527
        frame "Single Event Latchup", Default {
        }
        frame "Single Event Transient" {
        }
      }
      n194 = Build Array("Run Number" ("name"), "DUT" ("element"), "Ion" ("element"), "Board Number" ("element"), "Effective LET" ("element"), "Test Type" ("element")) -> (w526:string[])
      n195 = Build Array(w533, w532, w531, w530, w529, w527) -> (w525:string[])
      n196 = Build Array(w526, w525) -> (w514:string[][])
      n197 = Build Path(base path=w479, name or relative path="RunData_Params.csv") -> (appended path=w520:path)
      n198 = call-poly <vilib>:"Write Delimited Spreadsheet.vi"("file path (dialog if empty)"=w520, "format (%s)"="%s" ("format (%.3f)"), "2D data"=w514, "error in (no error)"=w515, "transpose? (no:F)"=TRUE, "delimiter (\\t)"="," ("delimiter (\\t)")) -> ()  [unwired: 8 in, 2 out]
      n199 = List Folder(path=w479, pattern="*NULL.txt") -> (path out=w498:path, filenames=w499:string[], error out=w500:errorcluster)  [unwired: 2 in, 1 out]
      n200 = for {
        tunnel: [w615] -> w510
        tunnel: w498 -> [w615]
        tunnel: w499 -> [w617] mode=indexing
        shift-right: [w618] -> w501
        shift-left: w500 -> [w619]
        n201 = Build Path(base path=w615, name or relative path=w617) -> (appended path=w616:path)
        n202 = Delete(path (use dialog)=w616, error in=w619) -> (error out=w618:errorcluster)  [unwired: 3 in, 2 out]
      }
      n203 = Get Date/Time String(date format (0)=enum16{"short", "long", "abbreviated"}."short", seconds (now)=w480, want seconds? (F)=TRUE) -> (date string=w504:string, time string=w503:string)
      n204 = Concatenate Strings(w504, "_" ("string"), w503) -> (w505:string)
      n205 = Strip Path(path=w510) -> (name=w496:string)  [unwired: 1 out]
      n206 = Build Path(base path=w510, name or relative path="BeginRecordTimeStamp.txt") -> (appended path=w511:path)
      n207 = Concatenate Strings(w496, "_DCPOWER_COPYFOLDER" ("name or relative path")) -> (w497:string)
      n208 = Open/Create/Replace File(file path (use dialog)=w511, error in=w501, operation (0:open)=T11."open or create", access (0:read/write)=enum16{"read/write", "read-only", "write-only"}."read/write") -> (refnum out=w506:refnum<file>, error out=w502:errorcluster)  [unwired: 2 in, 1 out]
      n209 = Build Path(base path=w510, name or relative path=w497) -> (appended path=w490:path)
      n210 = Write to Text File(file (use dialog)=w506, text=w505, error in=w502) -> (refnum out=w508:refnum<file>, error out=w507:errorcluster)  [unwired: 1 in, 1 out]
      n211 = Close File(refnum=w508, error in=w507) -> (error out=w509:errorcluster)  [unwired: 1 out]
      n212 = Create Folder(path (use dialog)=w490, error in=w509) -> (created path=w494:path, error out=w491:errorcluster)  [unwired: 1 in, 1 out]
      n213 = List Folder(path=w510, error in=w491) -> (path out=w492:path, filenames=w493:string[], error out=w495:errorcluster)  [unwired: 2 in, 1 out]
      n214 = for {
        tunnel: w492 -> [w625]
        tunnel: w493 -> [w624] mode=indexing
        tunnel: w494 -> [w620]
        shift-right: [w627] -> w481
        shift-left: w495 -> [w621]
        tunnel: [w620] -> _
        n215 = Build Path(base path=w625, name or relative path=w624) -> (appended path=w622:path)
        n216 = Build Path(base path=w620, name or relative path=w624) -> (appended path=w623:path)
        n217 = Copy(8:w621, 9:TRUE ("overwrite (F)"), 10:w623, 11:w622) -> (0:w627:errorcluster)  [unwired: 1 in, 2 out]
      }
    }
  }
  "DCPowerInformationClusterArray_Output" <- w33
  "VISAPowerInfoInputOutput" <- w35
  "Run Data SubPanel Output" <- w37
  "Oscilloscope Info Array Output" <- w41
  "Data Was Collected?" <- w30
  "DCPowerInfoArray" <- w29
  "OscilloscopeInfoArray" <- w18
  "RFSourceInfoArray" <- w17
  "RF Subpanel Output" <- w39
  "error out" <- w2
